vi "ClusterEscala.vi"() -> ()   [LabVIEW 2020]
panel:
  out "Cluster 2":T1 {"N/m^2/V" scale=0.0..50.0; "l/Seg/V" scale=0.0..50.0; "C°/V" scale=0.0..100.0}
  out "resultados":cluster{dbl, dbl, dbl}
  in  "Cluster":T2
  # "C° /V"
  # "l/seg/V"
  # "N/m^2/V"
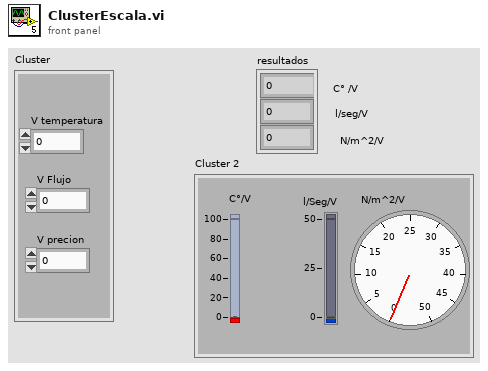
[diagram p1: front panel]
types:
  T1 = cluster{"C°/V":dbl, "l/Seg/V":dbl, "N/m^2/V":dbl}
  T2 = cluster{"V temperatura":dbl, "V Flujo":dbl, "V precion":dbl}
  T3 = cluster{"C°/V":dbl, "l/seg/V":dbl, "N/m^2/V":dbl}
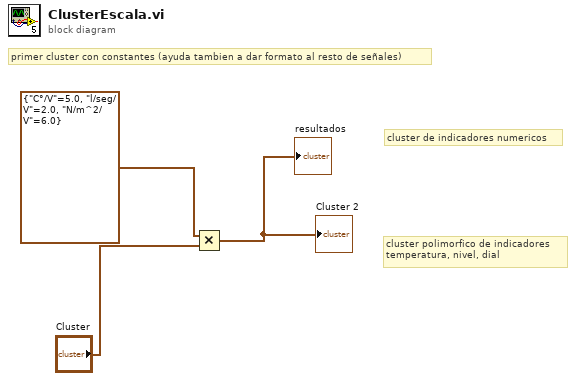
[diagram p0: block diagram]
diagram:
  # "cluster de indicadores numericos"
  # "cluster polimorfico de indicadores\ntemperatura, nivel, dial"
  # "primer cluster con constantes (ayuda tambien a dar formato al resto de señales)"
  n1 = Multiply(x=T3 {"C°/V"=5.0, "l/seg/V"=2.0, "N/m^2/V"=6.0}, y="Cluster") -> (x*y=→"resultados" →"Cluster 2":cluster{dbl, dbl, dbl})
